vi "error table.vi"(0 "connection refrence":T1, 1 "table":string, 2 "cam error":errorcluster, 3 "Sensor Error":errorcluster, 4 "error in":errorcluster) -> (14 "connection reference out":T1, 17 "error out":errorcluster)   [LabVIEW 2019]
uses:
  <vilib>/addons/database/Connection.llb/Conn ObjectReference.ctl
  <vilib>/addons/database/Auxilliary.llb/DB Tools Format Datetime String (Time Stamp).vi
  <vilib>/addons/database/NI_Database_API.lvlib
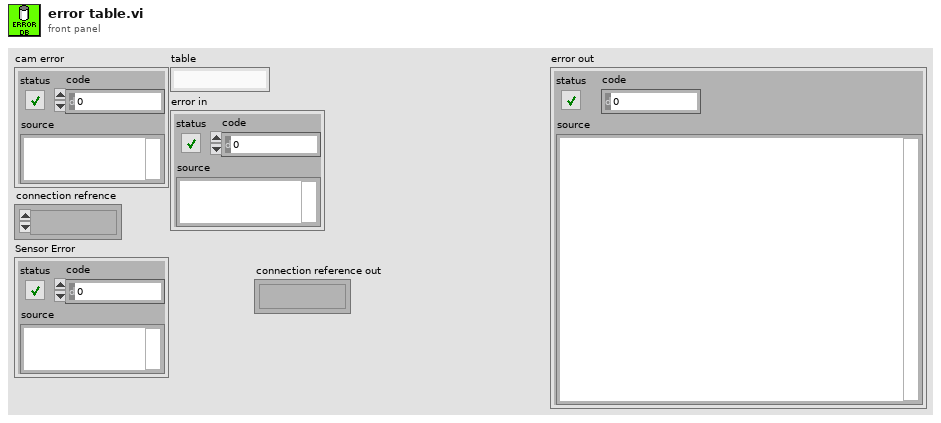
[diagram p1: front panel]
types:
  T1 = typedef "NI_Database_API.lvlib/Conn ObjectReference.ctl" = refnum<k1>
  T2 = cluster{"date/time string":string, string, string}
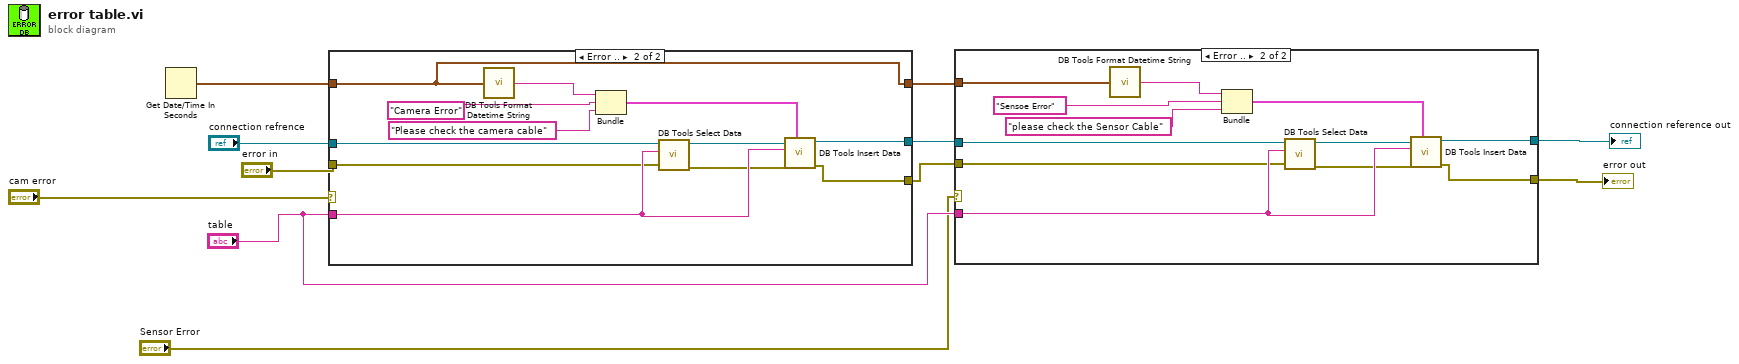
[diagram p0: block diagram]
diagram:
  n1 = Get Date/Time In Seconds() -> (seconds since 1Jan1904=w11:timestamp)
  n2 = case shown="Error .." "cam error" {
    tunnel: w11 -> [w12 w15]
    tunnel: "connection refrence" -> [w14 w25]
    tunnel: "table" -> [_ w22]
    tunnel: "error in" -> [w13 w21]
    tunnel: [w14 w19] -> w6
    tunnel: [w13 w18] -> w7
    tunnel: [w12 w15] -> w5
    frame No Error {
    }
    frame Error {
      n3 = call-poly <vilib>:"DB Tools Format Datetime String.vi"("time stamp"=w15) -> ("date/time string"=w26:string)
      n4 = Bundle("date/time string"=w26, "Camera Error", "Please check the camera cable") -> (w23:T2)  [unwired: 1 in]
      n5 = call <vilib>:"DB Tools Select Data.vi"("error in (no error)"=w21, "table"=w22, "connection reference"=w25) -> ("error out"=w20:errorcluster, "connection reference out"=w24:T1)  [unwired: 3 in, 1 out]
      n6 = call <vilib>:"DB Tools Insert Data.vi"("data"=w23, "error in (no error)"=w20, "table"=w22, "connection reference"=w24) -> ("error out"=w18:errorcluster, "connection reference out"=w19:T1)  [unwired: 6 in]
    }
  }
  n7 = case shown="Error .." "Sensor Error" {
    tunnel: w5 -> [_ w40]
    tunnel: w6 -> [w28 w37]
    tunnel: "table" -> [_ w34]
    tunnel: w7 -> [w27 w33]
    tunnel: [w28 w31] -> w1
    tunnel: [w27 w30] -> w2
    frame No Error {
    }
    frame Error {
      n8 = call-poly <vilib>:"DB Tools Format Datetime String.vi"("time stamp"=w40) -> ("date/time string"=w39:string)
      n9 = Bundle("date/time string"=w39, "Sensoe Error", "please check the Sensor Cable") -> (w35:T2)  [unwired: 1 in]
      n10 = call <vilib>:"DB Tools Select Data.vi"("error in (no error)"=w33, "table"=w34, "connection reference"=w37) -> ("error out"=w32:errorcluster, "connection reference out"=w36:T1)  [unwired: 3 in, 1 out]
      n11 = call <vilib>:"DB Tools Insert Data.vi"("data"=w35, "error in (no error)"=w32, "table"=w34, "connection reference"=w36) -> ("error out"=w30:errorcluster, "connection reference out"=w31:T1)  [unwired: 6 in]
    }
  }
  "error out" <- w2
  "connection reference out" <- w1
